vi "Untitled 1.vi"(8 "stop":bool, 11 "Position":i32) -> (3 "Sensor Reading":i32(graph))   [LabVIEW 2013]
panel:
  out "Handle":u32
  out "FT_Status 2":u32(ring) items=["FT_OK", "FT_INVALID_HANDLE", "FT_DEVICE_NOT_FOUND", "FT_DEVICE_NOT_OPENED", "FT_IO_ERROR", "FT_INSUFFICIENT_RESOURCES", "FT_INVALID_PARAMETER", "FT_INVALID_BAUD_RATE", "FT_DEVICE_NOT_OPENED_FOR_ERASE", "FT_DEVICE_NOT_OPENED_FOR_WRITE", "FT_FAILED_TO_WRITE_DEVICE", "FT_EEPROM_READ_FAILED", "FT_EEPROM_WRITE_FAILED", "FT_EEPROM_ERASE_FAILED", "FT_EEPROM_NOT_PRESENT", "FT_EEPROM_NOT_PROGRAMMED", "FT_INVALID_ARGS", "FT_NOT_SUPPORTED", "FT_OTHER_ERROR"]
  out "FT_Status":u32(ring) items=["FT_OK", "FT_INVALID_HANDLE", "FT_DEVICE_NOT_FOUND", "FT_DEVICE_NOT_OPENED", "FT_IO_ERROR", "FT_INSUFFICIENT_RESOURCES", "FT_INVALID_PARAMETER", "FT_INVALID_BAUD_RATE", "FT_DEVICE_NOT_OPENED_FOR_ERASE", "FT_DEVICE_NOT_OPENED_FOR_WRITE", "FT_FAILED_TO_WRITE_DEVICE", "FT_EEPROM_READ_FAILED", "FT_EEPROM_WRITE_FAILED", "FT_EEPROM_ERASE_FAILED", "FT_EEPROM_NOT_PRESENT", "FT_EEPROM_NOT_PROGRAMMED", "FT_INVALID_ARGS", "FT_NOT_SUPPORTED", "FT_OTHER_ERROR"]
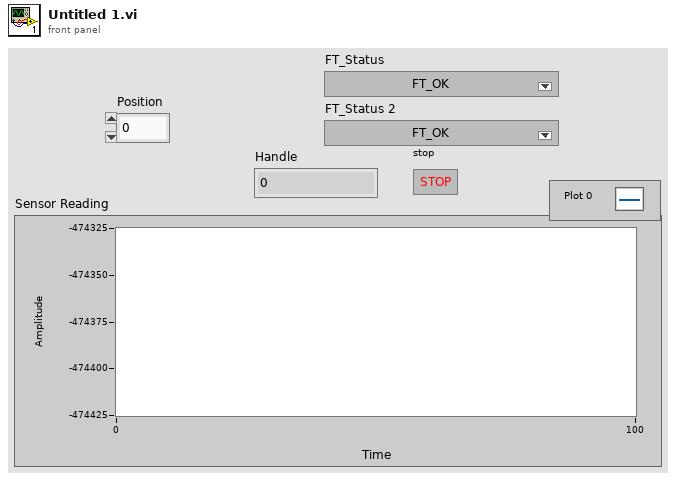
[diagram p1: front panel]
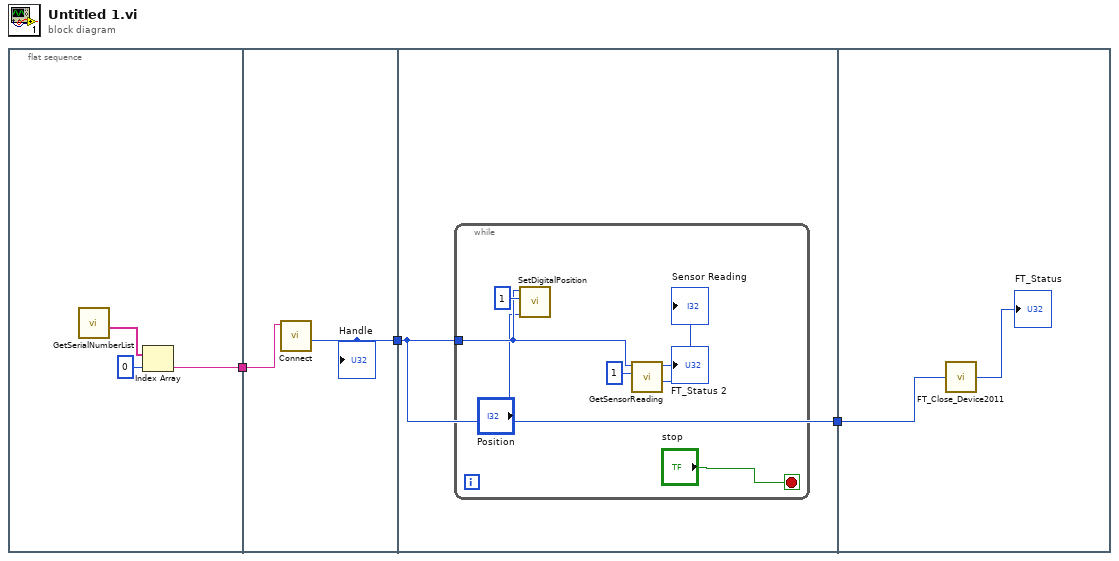
[diagram p0: block diagram]
diagram:
  n1 = flat-sequence {
    tunnel: [w4] -> w3
    tunnel: w3 -> [w8]
    tunnel: [w7] -> w2
    tunnel: w2 -> [w9]
    tunnel: [w9] -> w1
    tunnel: w1 -> [w17]
    frame #0 {
      n2 = call "GetSerialNumberList.vi"() -> ("C400 Serial Number Array"=w5:string[])  [unwired: 11 in]
      n3 = Index Array(array=w5, index=0) -> (element=w4:string)
    }
    frame #1 {
      n4 = call "Connect.vi"("Device Serial Number"=w8) -> ("Handle"=w7:u32)  [unwired: 9 in, 1 out]
      "Handle" <- w7
    }
    frame #2 {
      n5 = while {
        tunnel: w9 -> [w11]
        stop <- "stop" stop-if-true
        n6 = call "SetDigitalPosition.vi"("Position"="Position", "Controller Channel"=1, "Handle"=w11) -> ()  [unwired: 8 in, 1 out]
        n7 = call "GetSensorReading.vi"("Handle"=w11, "Controller Channel"=1) -> ("FT_Status"=→"FT_Status 2":u32, "Sensor Reading"=→"Sensor Reading":i32)  [unwired: 7 in]
      }
    }
    frame #3 {
      n8 = call "FT_Close_Device2011.vi"("Handle"=w17) -> ("FT_Status"=→"FT_Status":u32)
    }
  }
